vi "niRFUtil WFM Apply Frequency Offset.vi"(0 "Waveform In":T1 {"y" format="%.2f"; "dx" format="%^.2e"; "x0" format="%^.2e"}, 11 "error in (no error)":errorcluster, 12 "Initial Phase (deg)":sgl format="%.2f", 13 "Offset (Hz)":sgl format="%^.2e") -> (4 "Waveform Out":T1 {"y" format="%.2f"; "dx" format="%^.2e"; "x0" format="%^.2e"}, 15 "error out":errorcluster)   [LabVIEW 2015, in "niRFUtil.lvlib"]
doc: "(c) Copyright 2006, National Instruments, Inc. This VI may not be duplicated, sold, or distributed without written consent from National Instruments."
uses:
  niRFUtil.lvlib
  Includes/niRFUtil INC Complex Waveform.ctl
  Includes/niRFUtil INC Complex Array.ctl
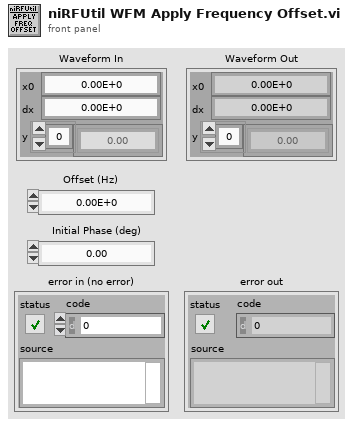
[diagram p1: front panel]
types:
  T1 = typedef "niRFUtil.lvlib/niRFUtil INC Complex Waveform.ctl" = cluster{"x0":dbl, "dx":dbl, "y":T2}
  T2 = typedef "niRFUtil.lvlib/niRFUtil INC Complex Array.ctl" = csg[]
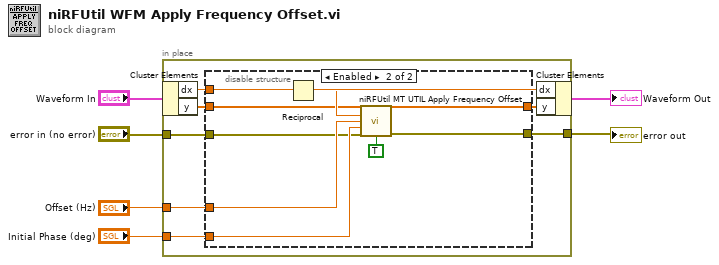
[diagram p0: block diagram]
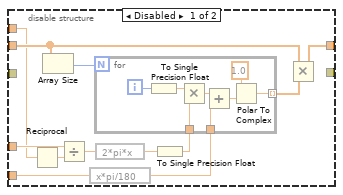
[diagram p2: hidden frame]
diagram:
  n1 = in-place {
    in-place-border: "Offset (Hz)" -> [w13]
    in-place-border: "Initial Phase (deg)" -> [w9]
    in-place-border: [w8] -> w2
    in-place-border: "error in (no error)" -> [w7]
    n2 = in-place-cluster #1("Waveform In") -> ("dx"=w11:dbl, "y"=w12:T2)
    n3 = disable-structure shown="Enabled" {
      disable-tunnel: w13 -> [w25 w41]
      disable-tunnel: w12 -> [w24 w38]
      disable-tunnel: w11 -> [w23 w40]
      disable-tunnel: [w22 w37] -> w10
      disable-tunnel: w9 -> [w15 w42]
      disable-tunnel: [_ w35] -> w8
      disable-tunnel: w7 -> [_ w34]
      frame Disabled {
        n4 = Reciprocal(x=w23) -> (1/x=w21:dbl)
        n5 = Array Size(array=w24) -> (size(s)=w20:i32)
        n6 = Divide(x=w25, y=w21) -> (x/y=w16:dbl)
        n7 = expression code="x*pi/180"(w15) -> (w14:sgl)
        n8 = expression code="2*pi*x"(w16) -> (w19:dbl)
        n9 = To Single Precision Float(number=w19) -> (single precision float=w17:sgl)
        n10 = for {
          N: w20 -> [_]
          tunnel: w17 -> [w32]
          tunnel: [w30] -> w18 mode=indexing
          tunnel: w14 -> [w28]
          i -> [w33]
          n11 = To Single Precision Float(number=w33) -> (single precision float=w31:sgl)
          n12 = Multiply(x=w31, y=w32) -> (x*y=w27:sgl)
          n13 = Add(x=w27, y=w28) -> (x+y=w26:sgl)
          n14 = Polar To Complex(1:w26, 2:sgl 1.0) -> (0:w30:csg)
        }
        n15 = Multiply(x=w24, y=w18) -> (x*y=w22:T2)
      }
      frame Enabled {
        n16 = Reciprocal(x=w40) -> (1/x=w39:dbl)
        n17 = call "niRFUtil MT UTIL Apply Frequency Offset.vi"("Signal In"=w38, "Rate (S/s)"=w39, "Freq Offset (Hz)"=w41, "Initial Phase (deg)"=w42, "error in (no error)"=w34, "Reset? (T)"=TRUE) -> ("Signal Out"=w37:T2, "error out"=w35:errorcluster)  [unwired: 8 in]
      }
    }
    n18 = in-place-cluster #1("dx"=w11, "y"=w10) -> (→"Waveform Out":T1)
  }
  "error out" <- w2
